vi "AddRefDevice.vi"(0 "reference in":refnum<class "Devices Controller.lvclass">, 2 "details":T2, 3 "Device Type":T1=enum."k4b2", 5 "error in (no error)":errorcluster) -> (14 "reference out":refnum<class "Devices Controller.lvclass">, 17 "index":i32, 19 "error out":errorcluster)   [LabVIEW 2015, in "Devices Controller.lvclass"]
uses:
  Devices Controller.lvclass
  deviceType.ctl
  APP/k5_class/k5.lvclass
  APP/peapod_class/peapod.lvclass
  APP/k4b2_class/k4b2.lvclass
  APP/fitmate_class/fitmate.lvclass
  APP/cpet_class/cpet.lvclass
  APP/rmr_class/rmr.lvclass
  APP/bb-pft_class/bb-pft.lvclass
  APP/bodpod_class/bodpod.lvclass
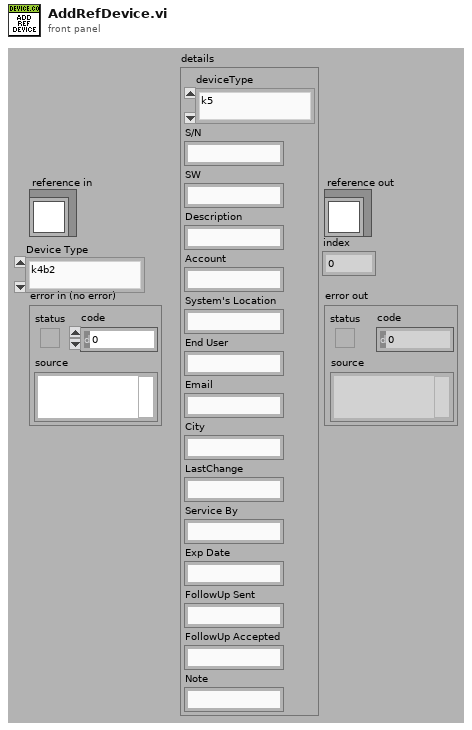
[diagram p1: front panel]
types:
  T1 = typedef "Devices Controller.lvclass/deviceType.ctl" = enum16{"k5", "k4b2", "fitmate", "cpet", "rmr", "bodyBoxPft", "bp", "pp"}
  T2 = cluster{"deviceType":T1, "S/N":string, "SW":string, "Description":string, "Account":string, "System's Location":string, "End User":string, "Email":string, "City":string, "LastChange":string, "Service By":string, "Exp Date":string, "FollowUp Sent":string, "FollowUp Accepted":string, "Note":string}
  T3 = cluster{"deviceType":T1, "S/N":string, "SW":string, "Description":string, "Account":string, "System's Location":string, "End User":string, "Email":string, "City":string, "FollowUp Sent":string, "FollowUp Accepted":string, "Note":string}
  T4 = typedef "Devices Controller.lvclass/ObjectAttributesRef.ctl" = refnum<data-value>
  T5 = typedef "Devices Controller.lvclass/ObjectAttributes.ctl" = cluster{"MyAttribute":dbl, "file_controller_ref":refnum<class "File Controller.lvclass">, "data":string[][][], "devices_refs":cluster{"k4b2_refs":refnum<class "k4b2.lvclass">[], "rmr_refs":refnum<class "rmr.lvclass">[], "bod_pod_refs":refnum<class "bodpod.lvclass">[], "cpet_refs":refnum<class "cpet.lvclass">[], "fitmate_refs":refnum<class "fitmate.lvclass">[], "pea_pod_refs":refnum<class "peapod.lvclass">[], "k5_refs":refnum<class "k5.lvclass">[], "bb-pft_refs":refnum<class "bb-pft.lvclass">[]}}
  T6 = cluster{"k4b2_refs":refnum<class "k4b2.lvclass">[], "rmr_refs":refnum<class "rmr.lvclass">[], "bod_pod_refs":refnum<class "bodpod.lvclass">[], "cpet_refs":refnum<class "cpet.lvclass">[], "fitmate_refs":refnum<class "fitmate.lvclass">[], "pea_pod_refs":refnum<class "peapod.lvclass">[], "k5_refs":refnum<class "k5.lvclass">[], "bb-pft_refs":refnum<class "bb-pft.lvclass">[]}
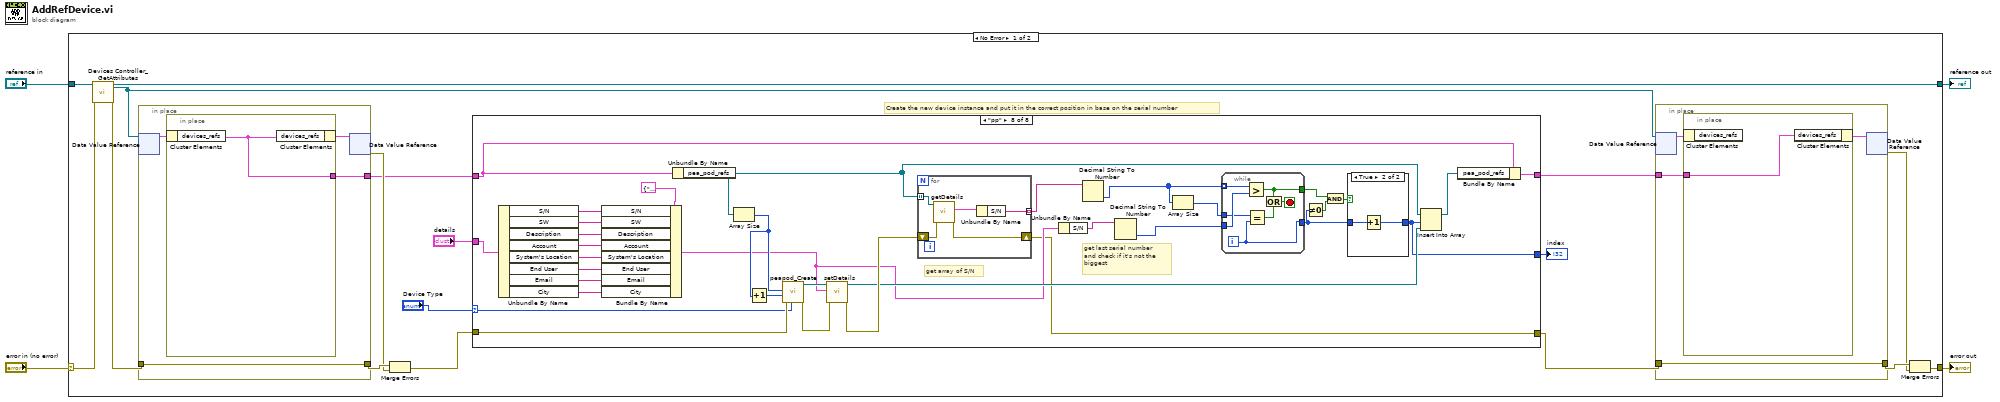
[diagram p0: block diagram]
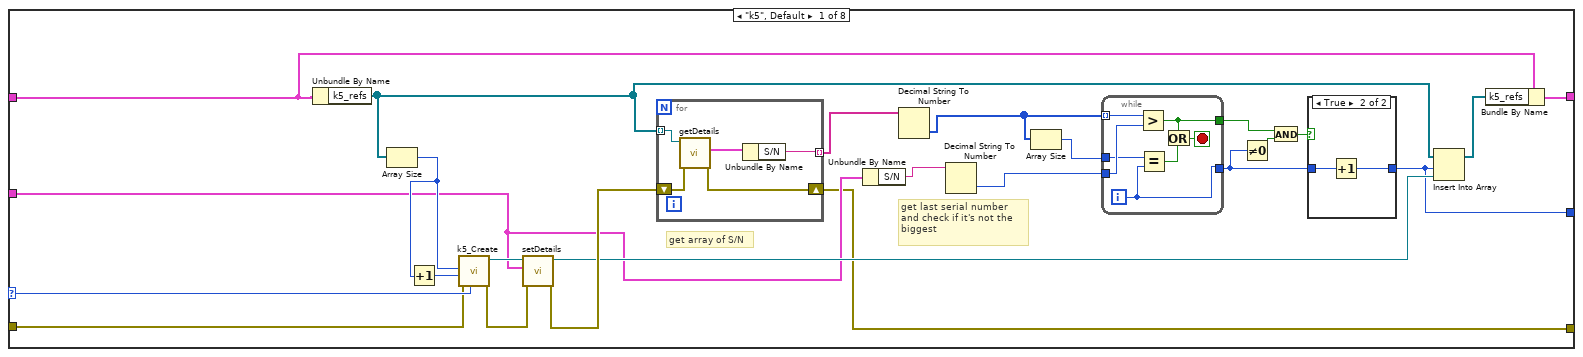
[diagram p2: hidden frame]
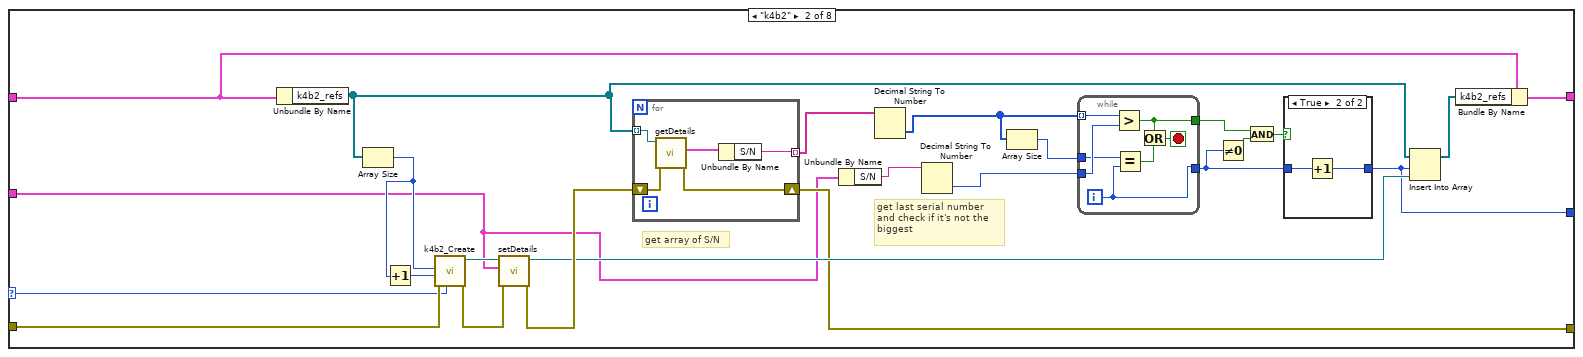
[diagram p4: hidden frame]
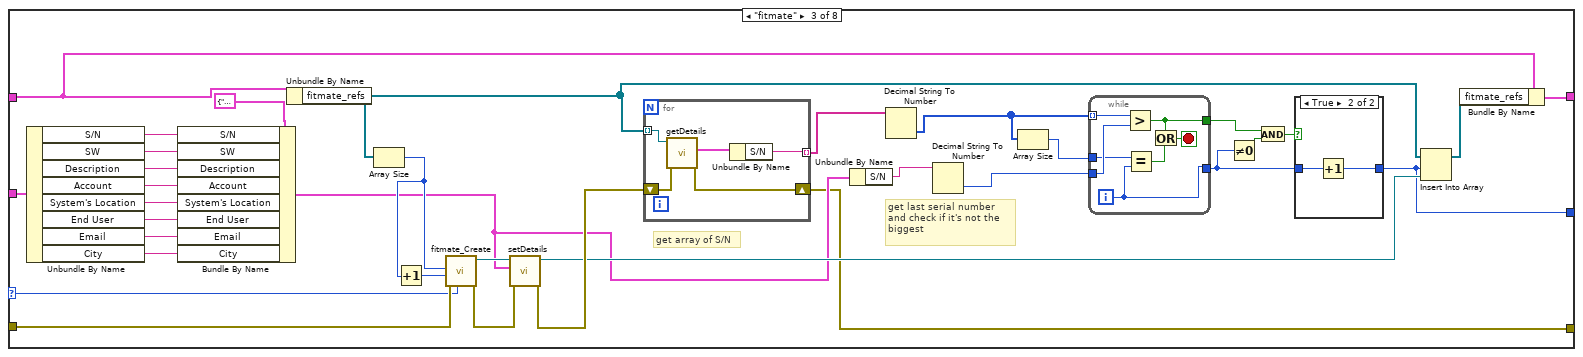
[diagram p6: hidden frame]
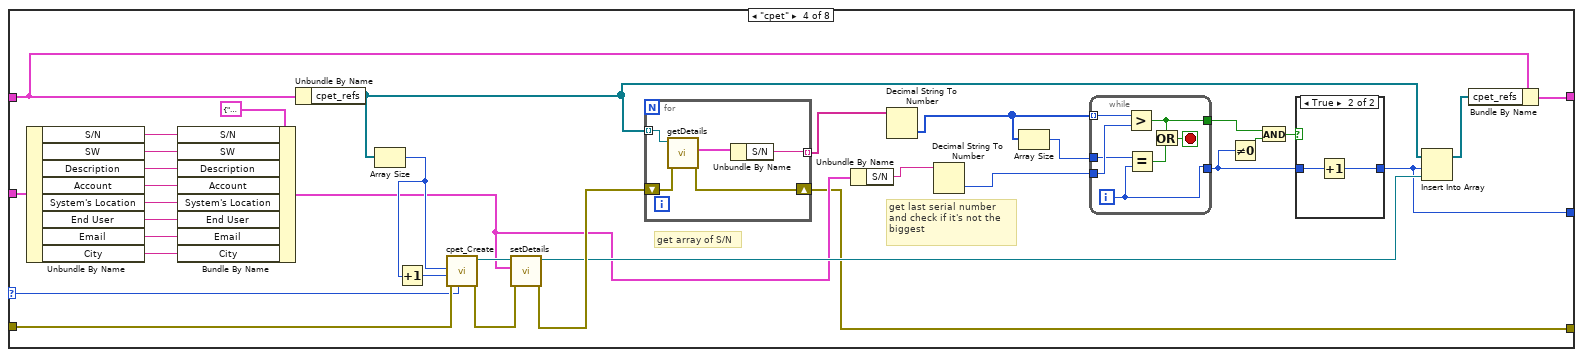
[diagram p8: hidden frame]
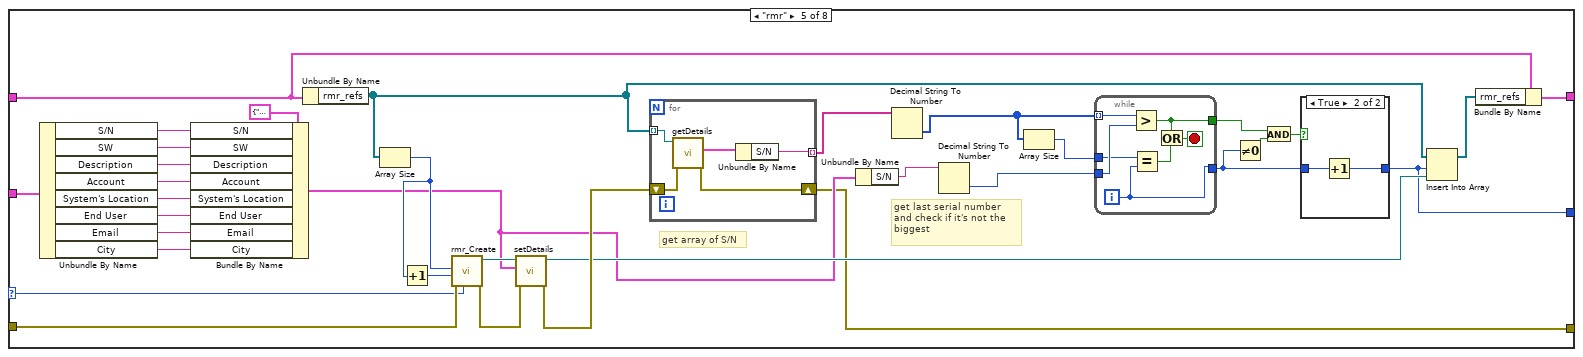
[diagram p10: hidden frame]
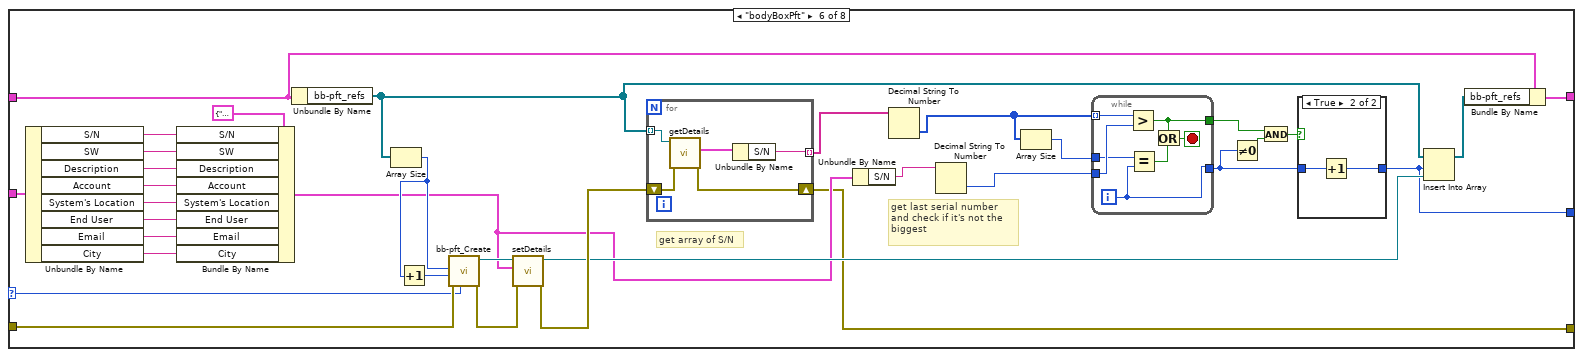
[diagram p12: hidden frame]
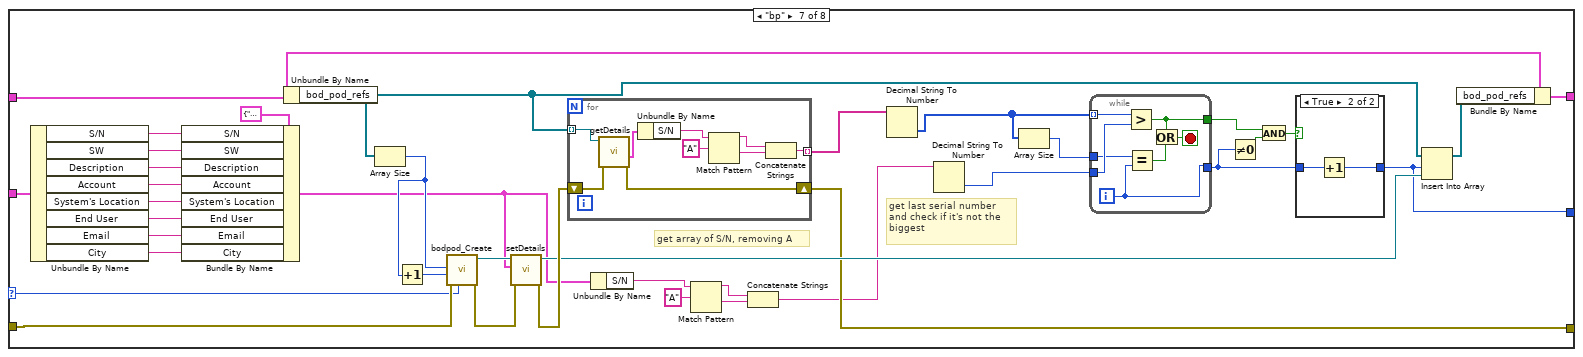
[diagram p14: hidden frame]
diagram:
  n1 = case shown="No Error" "error in (no error)" {
    selector: "error in (no error)" -> [w19 w413]
    tunnel: [w9 w413] -> w3
    tunnel: [w20 w412] -> w1
    tunnel: "reference in" -> [w21 w412]
    frame No Error {
      # "Create the new device instance and put it in the correct position in base on the serial number"
      n2 = call "Devices Controller_GetAttributes.vi"("reference in"=w21, "error in (no error)"=w19) -> ("reference out"=w20:refnum<class "Devices Controller.lvclass">, "attributes ref"=w13:T4, "error out"=w18:errorcluster)  [unwired: 14 in, 1 out]
      n3 = in-place {
        in-place-border: w18 -> [w408]
        in-place-border: [w408] -> w17
        in-place-border: [w407] -> w14
        n4 = in-place-dvr #1(w13) -> (w409:T5)  [unwired: 1 out]
        n5 = in-place {
          in-place-border: [w411] -> w407
          n6 = in-place-cluster #2(w409) -> ("devices_refs"=w411:T6)
          n7 = in-place-cluster #2("devices_refs"=w411) -> (w410:T5)
        }
        n8 = in-place-dvr #1(w410) -> (w16:errorcluster)  [unwired: 1 out]
      }
      n9 = Merge Errors(w17, w16) -> (w6:errorcluster)
      n10 = case shown="\"pp\"" "Device Type" {
        selector: "Device Type" -> [w42 w68 w110 w159 w206 w254 w309 w359]
        tunnel: w14 -> [w50 w72 w108 w157 w209 w258 w311 w368]
        tunnel: [w49 w71 w105 w154 w203 w252 w306 w367] -> w12
        tunnel: w6 -> [w41 w69 w111 w160 w208 w257 w312 w370]
        tunnel: "details" -> [w36 w67 w129 w178 w227 w276 w329 w382]
        tunnel: [w27 w66 w106 w155 w204 w253 w307 w360] -> w7
        tunnel: [w34 w70 w107 w156 w205 w255 w308 w366] -> w5
        frame "k5", Default {
          # "get last serial number\nand check if it's not the \nbiggest"
          # "get array of S/N"
          n11 = Unbundle By Name(w50) -> ("k5_refs"=w38:refnum<class "k5.lvclass">[])
          n12 = Array Size(array=w38) -> (size(s)=w43:i32)
          n13 = Increment(x=w43) -> (x+1=w45:i32)
          n14 = call "k5_Create.vi"("deviceType"=w42, "error in (no error)"=w41, "dim"=w45, "index"=w43) -> ("error out"=w40:errorcluster, "reference out"=w44:refnum<class "k5.lvclass">)  [unwired: 6 in]
          n15 = call "setDetails.vi"("error in (no error)"=w40, "details"=w36, "reference in"=w44) -> ("error out"=w39:errorcluster, "reference out"=w37:refnum<class "k5.lvclass">)  [unwired: 7 in]
          n16 = for {
            tunnel: w38 -> [w63] mode=indexing
            shift-right: [w64] -> w34
            shift-left: w39 -> [w65]
            tunnel: [w61] -> w48 mode=indexing
            n17 = call "getDetails.vi"("error in (no error)"=w65, "reference in"=w63) -> ("error out"=w64:errorcluster, "details"=w62:T2)  [unwired: 7 in, 1 out]
            n18 = Unbundle By Name(w62) -> ("S/N"=w61:string)
          }
          n19 = Unbundle By Name(w36) -> ("S/N"=w35:string)
          n20 = Decimal String To Number(string=w48) -> (number=w33:i32[])  [unwired: 2 in, 1 out]
          n21 = Decimal String To Number(string=w35) -> (number=w47:i32)  [unwired: 2 in, 1 out]
          n22 = Array Size(array=w33) -> (size(s)=w32:i32)
          n23 = while {
            tunnel: w33 -> [w60] mode=indexing
            tunnel: w47 -> [w59]
            tunnel: [w58] -> w28
            tunnel: w32 -> [w57]
            tunnel: [w54] -> w30
            i -> [w58]
            stop <- w55 stop-if-true
            n24 = Greater?(x=w60, y=w59) -> (0:w54:bool)
            n25 = Equal?(x=w57, y=w58) -> (x = y?=w56:bool)
            n26 = Or(x=w54, y=w56) -> (x .or. y?=w55:bool)
          }
          n27 = Not Equal To 0?(x=w28) -> (x != 0?=w31:bool)
          n28 = And(x=w30, y=w31) -> (x .and. y?=w29:bool)
          n29 = case shown="True" w29 {
            tunnel: w28 -> [w51 w53]
            tunnel: [w51 w52] -> w27
            frame False {
            }
            frame True {
              n30 = Increment(x=w53) -> (x+1=w52:i32)
            }
          }
          n31 = Insert Into Array(array=w38, index=w27, new element=w37) -> (w46:refnum<class "k5.lvclass">[])
          n32 = Bundle By Name(cluster=w50, "k5_refs"=w46) -> (w49:T6)
        }
        frame "k4b2" {
          # "get last serial number\nand check if it's not the \nbiggest"
          # "get array of S/N"
          n33 = Unbundle By Name(w72) -> ("k4b2_refs"=w81:refnum<class "k4b2.lvclass">[])
          n34 = Array Size(array=w81) -> (size(s)=w84:i32)
          n35 = Increment(x=w84) -> (x+1=w86:i32)
          n36 = call "k4b2_Create.vi"("deviceType"=w68, "error in (no error)"=w69, "dim"=w86, "index"=w84) -> ("error out"=w83:errorcluster, "reference out"=w85:refnum<class "k4b2.lvclass">)  [unwired: 6 in]
          n37 = call "setDetails.vi"("error in (no error)"=w83, "details"=w67, "reference in"=w85) -> ("error out"=w82:errorcluster, "reference out"=w80:refnum<class "k4b2.lvclass">)  [unwired: 7 in]
          n38 = for {
            tunnel: w81 -> [w102] mode=indexing
            shift-right: [w103] -> w70
            shift-left: w82 -> [w104]
            tunnel: [w100] -> w89 mode=indexing
            n39 = call "getDetails.vi"("error in (no error)"=w104, "reference in"=w102) -> ("error out"=w103:errorcluster, "details"=w101:T2)  [unwired: 7 in, 1 out]
            n40 = Unbundle By Name(w101) -> ("S/N"=w100:string)
          }
          n41 = Unbundle By Name(w67) -> ("S/N"=w79:string)
          n42 = Decimal String To Number(string=w89) -> (number=w78:i32[])  [unwired: 2 in, 1 out]
          n43 = Decimal String To Number(string=w79) -> (number=w88:i32)  [unwired: 2 in, 1 out]
          n44 = Array Size(array=w78) -> (size(s)=w77:i32)
          n45 = while {
            tunnel: w78 -> [w99] mode=indexing
            tunnel: w88 -> [w98]
            tunnel: [w97] -> w73
            tunnel: w77 -> [w96]
            tunnel: [w93] -> w75
            i -> [w97]
            stop <- w94 stop-if-true
            n46 = Greater?(x=w99, y=w98) -> (0:w93:bool)
            n47 = Equal?(x=w96, y=w97) -> (x = y?=w95:bool)
            n48 = Or(x=w93, y=w95) -> (x .or. y?=w94:bool)
          }
          n49 = Not Equal To 0?(x=w73) -> (x != 0?=w76:bool)
          n50 = And(x=w75, y=w76) -> (x .and. y?=w74:bool)
          n51 = case shown="True" w74 {
            tunnel: w73 -> [w90 w92]
            tunnel: [w90 w91] -> w66
            frame False {
            }
            frame True {
              n52 = Increment(x=w92) -> (x+1=w91:i32)
            }
          }
          n53 = Insert Into Array(array=w81, index=w66, new element=w80) -> (w87:refnum<class "k4b2.lvclass">[])
          n54 = Bundle By Name(cluster=w72, "k4b2_refs"=w87) -> (w71:T6)
        }
        frame "fitmate" {
          # "get last serial number\nand check if it's not the \nbiggest"
          # "get array of S/N"
          n55 = Unbundle By Name(w129) -> ("S/N"=w138:string, "SW"=w137:string, "Description"=w136:string, "Account"=w135:string, "System's Location"=w134:string, "End User"=w133:string, "Email"=w132:string, "City"=w131:string)
          n56 = Bundle By Name(cluster=T3 {"deviceType"=enum."k5", "S/N"="", "SW"="", "Description"="", "Account"="", "System's Location"="", "End User"="", "Email"="", "City"="", "FollowUp Sent"="", "FollowUp Accepted"="", "Note"=""} ("details"), "S/N"=w138, "SW"=w137, "Description"=w136, "Account"=w135, "System's Location"=w134, "End User"=w133, "Email"=w132, "City"=w131) -> (w109:T3)
          n57 = Unbundle By Name(w108) -> ("fitmate_refs"=w120:refnum<class "fitmate.lvclass">[])
          n58 = Array Size(array=w120) -> (size(s)=w123:i32)
          n59 = Increment(x=w123) -> (x+1=w125:i32)
          n60 = call "fitmate_Create.vi"("deviceType"=w110, "error in (no error)"=w111, "dim"=w125, "index"=w123) -> ("error out"=w122:errorcluster, "reference out"=w124:refnum<class "fitmate.lvclass">)  [unwired: 6 in]
          n61 = call "setDetails.vi"("error in (no error)"=w122, "details"=w109, "reference in"=w124) -> ("error out"=w121:errorcluster, "reference out"=w119:refnum<class "fitmate.lvclass">)  [unwired: 7 in]
          n62 = for {
            tunnel: w120 -> [w151] mode=indexing
            shift-right: [w152] -> w107
            shift-left: w121 -> [w153]
            tunnel: [w149] -> w128 mode=indexing
            n63 = call "getDetails.vi"("error in (no error)"=w153, "reference in"=w151) -> ("error out"=w152:errorcluster, "details"=w150:T3)  [unwired: 7 in, 1 out]
            n64 = Unbundle By Name(w150) -> ("S/N"=w149:string)
          }
          n65 = Unbundle By Name(w109) -> ("S/N"=w118:string)
          n66 = Decimal String To Number(string=w128) -> (number=w117:i32[])  [unwired: 2 in, 1 out]
          n67 = Decimal String To Number(string=w118) -> (number=w127:i32)  [unwired: 2 in, 1 out]
          n68 = Array Size(array=w117) -> (size(s)=w116:i32)
          n69 = while {
            tunnel: w117 -> [w148] mode=indexing
            tunnel: w127 -> [w147]
            tunnel: [w146] -> w112
            tunnel: w116 -> [w145]
            tunnel: [w142] -> w114
            i -> [w146]
            stop <- w143 stop-if-true
            n70 = Greater?(x=w148, y=w147) -> (0:w142:bool)
            n71 = Equal?(x=w145, y=w146) -> (x = y?=w144:bool)
            n72 = Or(x=w142, y=w144) -> (x .or. y?=w143:bool)
          }
          n73 = Not Equal To 0?(x=w112) -> (x != 0?=w115:bool)
          n74 = And(x=w114, y=w115) -> (x .and. y?=w113:bool)
          n75 = case shown="True" w113 {
            tunnel: w112 -> [w139 w141]
            tunnel: [w139 w140] -> w106
            frame False {
            }
            frame True {
              n76 = Increment(x=w141) -> (x+1=w140:i32)
            }
          }
          n77 = Insert Into Array(array=w120, index=w106, new element=w119) -> (w126:refnum<class "fitmate.lvclass">[])
          n78 = Bundle By Name(cluster=w108, "fitmate_refs"=w126) -> (w105:T6)
        }
        frame "cpet" {
          # "get last serial number\nand check if it's not the \nbiggest"
          # "get array of S/N"
          n79 = Unbundle By Name(w178) -> ("S/N"=w187:string, "SW"=w186:string, "Description"=w185:string, "Account"=w184:string, "System's Location"=w183:string, "End User"=w182:string, "Email"=w181:string, "City"=w180:string)
          n80 = Bundle By Name(cluster=T3 {"deviceType"=enum."k5", "S/N"="", "SW"="", "Description"="", "Account"="", "System's Location"="", "End User"="", "Email"="", "City"="", "FollowUp Sent"="", "FollowUp Accepted"="", "Note"=""} ("details"), "S/N"=w187, "SW"=w186, "Description"=w185, "Account"=w184, "System's Location"=w183, "End User"=w182, "Email"=w181, "City"=w180) -> (w158:T3)
          n81 = Unbundle By Name(w157) -> ("cpet_refs"=w169:refnum<class "cpet.lvclass">[])
          n82 = Array Size(array=w169) -> (size(s)=w172:i32)
          n83 = Increment(x=w172) -> (x+1=w174:i32)
          n84 = call "cpet_Create.vi"("deviceType"=w159, "error in (no error)"=w160, "dim"=w174, "index"=w172) -> ("error out"=w171:errorcluster, "reference out"=w173:refnum<class "cpet.lvclass">)  [unwired: 6 in]
          n85 = call "setDetails.vi"("error in (no error)"=w171, "details"=w158, "reference in"=w173) -> ("error out"=w170:errorcluster, "reference out"=w168:refnum<class "cpet.lvclass">)  [unwired: 7 in]
          n86 = for {
            tunnel: w169 -> [w200] mode=indexing
            shift-right: [w201] -> w156
            shift-left: w170 -> [w202]
            tunnel: [w198] -> w177 mode=indexing
            n87 = call "getDetails.vi"("error in (no error)"=w202, "reference in"=w200) -> ("error out"=w201:errorcluster, "details"=w199:T3)  [unwired: 7 in, 1 out]
            n88 = Unbundle By Name(w199) -> ("S/N"=w198:string)
          }
          n89 = Unbundle By Name(w158) -> ("S/N"=w167:string)
          n90 = Decimal String To Number(string=w177) -> (number=w166:i32[])  [unwired: 2 in, 1 out]
          n91 = Decimal String To Number(string=w167) -> (number=w176:i32)  [unwired: 2 in, 1 out]
          n92 = Array Size(array=w166) -> (size(s)=w165:i32)
          n93 = while {
            tunnel: w166 -> [w197] mode=indexing
            tunnel: w176 -> [w196]
            tunnel: [w195] -> w161
            tunnel: w165 -> [w194]
            tunnel: [w191] -> w163
            i -> [w195]
            stop <- w192 stop-if-true
            n94 = Greater?(x=w197, y=w196) -> (0:w191:bool)
            n95 = Equal?(x=w194, y=w195) -> (x = y?=w193:bool)
            n96 = Or(x=w191, y=w193) -> (x .or. y?=w192:bool)
          }
          n97 = Not Equal To 0?(x=w161) -> (x != 0?=w164:bool)
          n98 = And(x=w163, y=w164) -> (x .and. y?=w162:bool)
          n99 = case shown="True" w162 {
            tunnel: w161 -> [w188 w190]
            tunnel: [w188 w189] -> w155
            frame False {
            }
            frame True {
              n100 = Increment(x=w190) -> (x+1=w189:i32)
            }
          }
          n101 = Insert Into Array(array=w169, index=w155, new element=w168) -> (w175:refnum<class "cpet.lvclass">[])
          n102 = Bundle By Name(cluster=w157, "cpet_refs"=w175) -> (w154:T6)
        }
        frame "rmr" {
          # "get last serial number\nand check if it's not the \nbiggest"
          # "get array of S/N"
          n103 = Unbundle By Name(w227) -> ("S/N"=w236:string, "SW"=w235:string, "Description"=w234:string, "Account"=w233:string, "System's Location"=w232:string, "End User"=w231:string, "Email"=w230:string, "City"=w229:string)
          n104 = Bundle By Name(cluster=T3 {"deviceType"=enum."k5", "S/N"="", "SW"="", "Description"="", "Account"="", "System's Location"="", "End User"="", "Email"="", "City"="", "FollowUp Sent"="", "FollowUp Accepted"="", "Note"=""} ("details"), "S/N"=w236, "SW"=w235, "Description"=w234, "Account"=w233, "System's Location"=w232, "End User"=w231, "Email"=w230, "City"=w229) -> (w207:T3)
          n105 = Unbundle By Name(w209) -> ("rmr_refs"=w218:refnum<class "rmr.lvclass">[])
          n106 = Array Size(array=w218) -> (size(s)=w221:i32)
          n107 = Increment(x=w221) -> (x+1=w223:i32)
          n108 = call "rmr_Create.vi"("deviceType"=w206, "error in (no error)"=w208, "dim"=w223, "index"=w221) -> ("error out"=w220:errorcluster, "reference out"=w222:refnum<class "rmr.lvclass">)  [unwired: 6 in]
          n109 = call "setDetails.vi"("error in (no error)"=w220, "details"=w207, "reference in"=w222) -> ("error out"=w219:errorcluster, "reference out"=w217:refnum<class "rmr.lvclass">)  [unwired: 7 in]
          n110 = for {
            tunnel: w218 -> [w249] mode=indexing
            shift-right: [w250] -> w205
            shift-left: w219 -> [w251]
            tunnel: [w247] -> w226 mode=indexing
            n111 = call "getDetails.vi"("error in (no error)"=w251, "reference in"=w249) -> ("error out"=w250:errorcluster, "details"=w248:T3)  [unwired: 7 in, 1 out]
            n112 = Unbundle By Name(w248) -> ("S/N"=w247:string)
          }
          n113 = Unbundle By Name(w207) -> ("S/N"=w216:string)
          n114 = Decimal String To Number(string=w226) -> (number=w215:i32[])  [unwired: 2 in, 1 out]
          n115 = Decimal String To Number(string=w216) -> (number=w225:i32)  [unwired: 2 in, 1 out]
          n116 = Array Size(array=w215) -> (size(s)=w214:i32)
          n117 = while {
            tunnel: w215 -> [w246] mode=indexing
            tunnel: w225 -> [w245]
            tunnel: [w244] -> w210
            tunnel: w214 -> [w243]
            tunnel: [w240] -> w212
            i -> [w244]
            stop <- w241 stop-if-true
            n118 = Greater?(x=w246, y=w245) -> (0:w240:bool)
            n119 = Equal?(x=w243, y=w244) -> (x = y?=w242:bool)
            n120 = Or(x=w240, y=w242) -> (x .or. y?=w241:bool)
          }
          n121 = Not Equal To 0?(x=w210) -> (x != 0?=w213:bool)
          n122 = And(x=w212, y=w213) -> (x .and. y?=w211:bool)
          n123 = case shown="True" w211 {
            tunnel: w210 -> [w237 w239]
            tunnel: [w237 w238] -> w204
            frame False {
            }
            frame True {
              n124 = Increment(x=w239) -> (x+1=w238:i32)
            }
          }
          n125 = Insert Into Array(array=w218, index=w204, new element=w217) -> (w224:refnum<class "rmr.lvclass">[])
          n126 = Bundle By Name(cluster=w209, "rmr_refs"=w224) -> (w203:T6)
        }
        frame "bodyBoxPft" {
          # "get last serial number\nand check if it's not the \nbiggest"
          # "get array of S/N"
          n127 = Unbundle By Name(w276) -> ("S/N"=w285:string, "SW"=w284:string, "Description"=w283:string, "Account"=w282:string, "System's Location"=w281:string, "End User"=w280:string, "Email"=w279:string, "City"=w278:string)
          n128 = Bundle By Name(cluster=T3 {"deviceType"=enum."k5", "S/N"="", "SW"="", "Description"="", "Account"="", "System's Location"="", "End User"="", "Email"="", "City"="", "FollowUp Sent"="", "FollowUp Accepted"="", "Note"=""} ("details"), "S/N"=w285, "SW"=w284, "Description"=w283, "Account"=w282, "System's Location"=w281, "End User"=w280, "Email"=w279, "City"=w278) -> (w256:T3)
          n129 = Unbundle By Name(w258) -> ("bb-pft_refs"=w267:refnum<class "bb-pft.lvclass">[])
          n130 = Array Size(array=w267) -> (size(s)=w270:i32)
          n131 = Increment(x=w270) -> (x+1=w272:i32)
          n132 = call "bb-pft_Create.vi"("deviceType"=w254, "error in (no error)"=w257, "dim"=w272, "index"=w270) -> ("error out"=w269:errorcluster, "reference out"=w271:refnum<class "bb-pft.lvclass">)  [unwired: 6 in]
          n133 = call "setDetails.vi"("error in (no error)"=w269, "details"=w256, "reference in"=w271) -> ("error out"=w268:errorcluster, "reference out"=w266:refnum<class "bb-pft.lvclass">)  [unwired: 7 in]
          n134 = for {
            tunnel: w267 -> [w298] mode=indexing
            shift-right: [w299] -> w255
            shift-left: w268 -> [w300]
            tunnel: [w296] -> w275 mode=indexing
            n135 = call "getDetails.vi"("error in (no error)"=w300, "reference in"=w298) -> ("error out"=w299:errorcluster, "details"=w297:T3)  [unwired: 7 in, 1 out]
            n136 = Unbundle By Name(w297) -> ("S/N"=w296:string)
          }
          n137 = Unbundle By Name(w256) -> ("S/N"=w265:string)
          n138 = Decimal String To Number(string=w275) -> (number=w264:i32[])  [unwired: 2 in, 1 out]
          n139 = Decimal String To Number(string=w265) -> (number=w274:i32)  [unwired: 2 in, 1 out]
          n140 = Array Size(array=w264) -> (size(s)=w263:i32)
          n141 = while {
            tunnel: w264 -> [w295] mode=indexing
            tunnel: w274 -> [w294]
            tunnel: [w293] -> w259
            tunnel: w263 -> [w292]
            tunnel: [w289] -> w261
            i -> [w293]
            stop <- w290 stop-if-true
            n142 = Greater?(x=w295, y=w294) -> (0:w289:bool)
            n143 = Equal?(x=w292, y=w293) -> (x = y?=w291:bool)
            n144 = Or(x=w289, y=w291) -> (x .or. y?=w290:bool)
          }
          n145 = Not Equal To 0?(x=w259) -> (x != 0?=w262:bool)
          n146 = And(x=w261, y=w262) -> (x .and. y?=w260:bool)
          n147 = case shown="True" w260 {
            tunnel: w259 -> [w286 w288]
            tunnel: [w286 w287] -> w253
            frame False {
            }
            frame True {
              n148 = Increment(x=w288) -> (x+1=w287:i32)
            }
          }
          n149 = Insert Into Array(array=w267, index=w253, new element=w266) -> (w273:refnum<class "bb-pft.lvclass">[])
          n150 = Bundle By Name(cluster=w258, "bb-pft_refs"=w273) -> (w252:T6)
        }
        frame "bp" {
          # "get last serial number\nand check if it's not the \nbiggest"
          # "get array of S/N, removing A"
          n151 = Unbundle By Name(w329) -> ("S/N"=w338:string, "SW"=w337:string, "Description"=w336:string, "Account"=w335:string, "System's Location"=w334:string, "End User"=w333:string, "Email"=w332:string, "City"=w331:string)
          n152 = Bundle By Name(cluster=T3 {"deviceType"=enum."k5", "S/N"="", "SW"="", "Description"="", "Account"="", "System's Location"="", "End User"="", "Email"="", "City"="", "FollowUp Sent"="", "FollowUp Accepted"="", "Note"=""} ("details"), "S/N"=w338, "SW"=w337, "Description"=w336, "Account"=w335, "System's Location"=w334, "End User"=w333, "Email"=w332, "City"=w331) -> (w310:T3)
          n153 = Unbundle By Name(w311) -> ("bod_pod_refs"=w320:refnum<class "bodpod.lvclass">[])
          n154 = Array Size(array=w320) -> (size(s)=w323:i32)
          n155 = Increment(x=w323) -> (x+1=w325:i32)
          n156 = call "bodpod_Create.vi"("deviceType"=w309, "error in (no error)"=w312, "dim"=w325, "index"=w323) -> ("error out"=w322:errorcluster, "reference out"=w324:refnum<class "bodpod.lvclass">)  [unwired: 6 in]
          n157 = call "setDetails.vi"("error in (no error)"=w322, "details"=w310, "reference in"=w324) -> ("error out"=w321:errorcluster, "reference out"=w319:refnum<class "bodpod.lvclass">)  [unwired: 7 in]
          n158 = for {
            tunnel: w320 -> [w355] mode=indexing
            shift-right: [w356] -> w308
            shift-left: w321 -> [w357]
            tunnel: [w349] -> w328 mode=indexing
            n159 = call "getDetails.vi"("error in (no error)"=w357, "reference in"=w355) -> ("error out"=w356:errorcluster, "details"=w354:T3)  [unwired: 7 in, 1 out]
            n160 = Unbundle By Name(w354) -> ("S/N"=w350:string)
            n161 = Match Pattern(string=w350, regular expression="A") -> (before substring=w352:string, after substring=w351:string)  [unwired: 1 in, 2 out]
            n162 = Concatenate Strings(w352, w351) -> (w349:string)
          }
          n163 = Unbundle By Name(w310) -> ("S/N"=w302:string)
          n164 = Match Pattern(string=w302, regular expression="A") -> (before substring=w304:string, after substring=w305:string)  [unwired: 1 in, 2 out]
          n165 = Concatenate Strings(w304, w305) -> (w301:string)
          n166 = Decimal String To Number(string=w328) -> (number=w318:i32[])  [unwired: 2 in, 1 out]
          n167 = Decimal String To Number(string=w301) -> (number=w327:i32)  [unwired: 2 in, 1 out]
          n168 = Array Size(array=w318) -> (size(s)=w317:i32)
          n169 = while {
            tunnel: w318 -> [w348] mode=indexing
            tunnel: w327 -> [w347]
            tunnel: [w346] -> w313
            tunnel: w317 -> [w345]
            tunnel: [w342] -> w315
            i -> [w346]
            stop <- w343 stop-if-true
            n170 = Greater?(x=w348, y=w347) -> (0:w342:bool)
            n171 = Equal?(x=w345, y=w346) -> (x = y?=w344:bool)
            n172 = Or(x=w342, y=w344) -> (x .or. y?=w343:bool)
          }
          n173 = Not Equal To 0?(x=w313) -> (x != 0?=w316:bool)
          n174 = And(x=w315, y=w316) -> (x .and. y?=w314:bool)
          n175 = case shown="True" w314 {
            tunnel: w313 -> [w339 w341]
            tunnel: [w339 w340] -> w307
            frame False {
            }
            frame True {
              n176 = Increment(x=w341) -> (x+1=w340:i32)
            }
          }
          n177 = Insert Into Array(array=w320, index=w307, new element=w319) -> (w326:refnum<class "bodpod.lvclass">[])
          n178 = Bundle By Name(cluster=w311, "bod_pod_refs"=w326) -> (w306:T6)
        }
        frame "pp" {
          # "get last serial number\nand check if it's not the \nbiggest"
          # "get array of S/N"
          n179 = Unbundle By Name(w382) -> ("S/N"=w391:string, "SW"=w390:string, "Description"=w389:string, "Account"=w388:string, "System's Location"=w387:string, "End User"=w386:string, "Email"=w385:string, "City"=w384:string)
          n180 = Bundle By Name(cluster=T3 {"deviceType"=enum."k5", "S/N"="", "SW"="", "Description"="", "Account"="", "System's Location"="", "End User"="", "Email"="", "City"="", "FollowUp Sent"="", "FollowUp Accepted"="", "Note"=""} ("details"), "S/N"=w391, "SW"=w390, "Description"=w389, "Account"=w388, "System's Location"=w387, "End User"=w386, "Email"=w385, "City"=w384) -> (w369:T3)
          n181 = Unbundle By Name(w368) -> ("pea_pod_refs"=w373:refnum<class "peapod.lvclass">[])
          n182 = Array Size(array=w373) -> (size(s)=w376:i32)
          n183 = Increment(x=w376) -> (x+1=w378:i32)
          n184 = call "peapod_Create.vi"("deviceType"=w359, "error in (no error)"=w370, "dim"=w378, "index"=w376) -> ("error out"=w375:errorcluster, "reference out"=w377:refnum<class "peapod.lvclass">)  [unwired: 6 in]
          n185 = call "setDetails.vi"("error in (no error)"=w375, "details"=w369, "reference in"=w377) -> ("error out"=w374:errorcluster, "reference out"=w372:refnum<class "peapod.lvclass">)  [unwired: 7 in]
          n186 = for {
            tunnel: w373 -> [w404] mode=indexing
            shift-right: [w405] -> w366
            shift-left: w374 -> [w406]
            tunnel: [w402] -> w381 mode=indexing
            n187 = call "getDetails.vi"("error in (no error)"=w406, "reference in"=w404) -> ("error out"=w405:errorcluster, "details"=w403:T3)  [unwired: 7 in, 1 out]
            n188 = Unbundle By Name(w403) -> ("S/N"=w402:string)
          }
          n189 = Unbundle By Name(w369) -> ("S/N"=w371:string)
          n190 = Decimal String To Number(string=w381) -> (number=w365:i32[])  [unwired: 2 in, 1 out]
          n191 = Decimal String To Number(string=w371) -> (number=w380:i32)  [unwired: 2 in, 1 out]
          n192 = Array Size(array=w365) -> (size(s)=w358:i32)
          n193 = while {
            tunnel: w365 -> [w401] mode=indexing
            tunnel: w380 -> [w400]
            tunnel: [w399] -> w361
            tunnel: w358 -> [w398]
            tunnel: [w395] -> w362
            i -> [w399]
            stop <- w396 stop-if-true
            n194 = Greater?(x=w401, y=w400) -> (0:w395:bool)
            n195 = Equal?(x=w398, y=w399) -> (x = y?=w397:bool)
            n196 = Or(x=w395, y=w397) -> (x .or. y?=w396:bool)
          }
          n197 = Not Equal To 0?(x=w361) -> (x != 0?=w364:bool)
          n198 = And(x=w362, y=w364) -> (x .and. y?=w363:bool)
          n199 = case shown="True" w363 {
            tunnel: [w392 w394] -> w360
            tunnel: w361 -> [w392 w393]
            frame False {
            }
            frame True {
              n200 = Increment(x=w393) -> (x+1=w394:i32)
            }
          }
          n201 = Insert Into Array(array=w373, index=w360, new element=w372) -> (w379:refnum<class "peapod.lvclass">[])
          n202 = Bundle By Name(cluster=w368, "pea_pod_refs"=w379) -> (w367:T6)
        }
      }
      "index" <- w7
      n203 = in-place {
        in-place-border: w5 -> [w23]
        in-place-border: [w23] -> w11
        in-place-border: w12 -> [w22]
        n204 = in-place-dvr #3(w13) -> (w24:T5)  [unwired: 1 out]
        n205 = in-place {
          in-place-border: w22 -> [w26]
          n206 = in-place-cluster #4(w24) -> ()  [unwired: 1 out]
          n207 = in-place-cluster #4("devices_refs"=w26) -> (w25:T5)
        }
        n208 = in-place-dvr #3(w25) -> (w10:errorcluster)  [unwired: 1 out]
      }
      n209 = Merge Errors(w11, w10) -> (w9:errorcluster)
    }
    frame Error {
    }
  }
  "error out" <- w3
  "reference out" <- w1
